vi "Temperature_Monitor.vi"() -> ()   [LabVIEW 2022 SP3]
panel:
  in  "?":bool
  out "?":string
  out "Temperature":dbl(slide) scale=-25.0..130.0
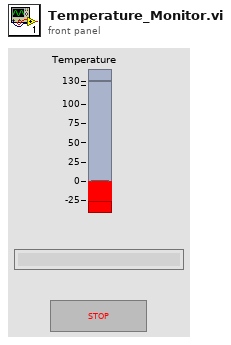
[diagram p1: front panel]
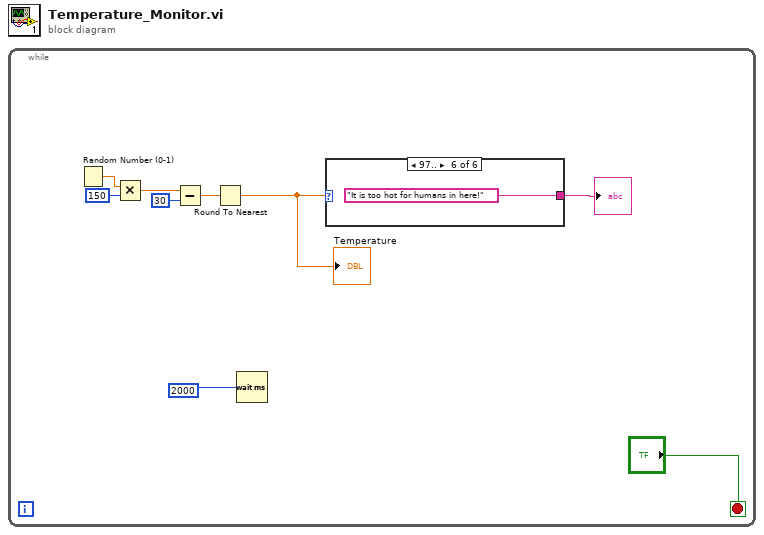
[diagram p0: block diagram]
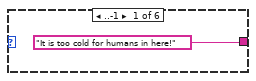
[diagram p2: hidden frame]
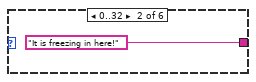
[diagram p3: hidden frame]
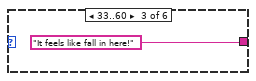
[diagram p4: hidden frame]
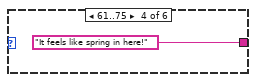
[diagram p5: hidden frame]
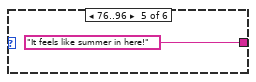
[diagram p6: hidden frame]
diagram:
  n1 = while {
    stop <- "?" stop-if-true
    n2 = Random Number (0-1)() -> (number: 0 to 1=w8:dbl)
    n3 = Multiply(x=w8, y=150) -> (x*y=w7:dbl)
    n4 = Subtract(x=w7, y=30) -> (x-y=w4:dbl)
    n5 = Round To Nearest(number=w4) -> (nearest integer value=w3:dbl)
    "Temperature" <- w3
    n6 = Wait (ms)(milliseconds to wait=2000) -> ()  [unwired: 1 out]
    n7 = case shown="97.." w3 {
      tunnel: ["It is too cold for humans in here!" "It is freezing in here!" "It feels like fall in here!" "It feels like spring in here!" "It feels like summer in here!" "It is too hot for humans in here!"] -> w5
      frame ..-1 {
      }
      frame 0..32 {
      }
      frame 33..60 {
      }
      frame 61..75 {
      }
      frame 76..96 {
      }
      frame 97.. {
      }
    }
    "?" <- w5
  }
